vi "Init AI.vi"(8 "error in (no error)":errorcluster, 10 "ADC #":T1=-1, 11 "Session in":refnum<class "Session.lvclass">) -> (0 "error out":errorcluster, 3 "Session out":refnum<class "Session.lvclass">)   [LabVIEW 2024, in "CTI.lvlib" / "Session.lvclass"]
uses:
  Session.lvclass
  ADC Number.ctl
  DeviceComms/DeviceComms.lvclass
  CTI.lvlib
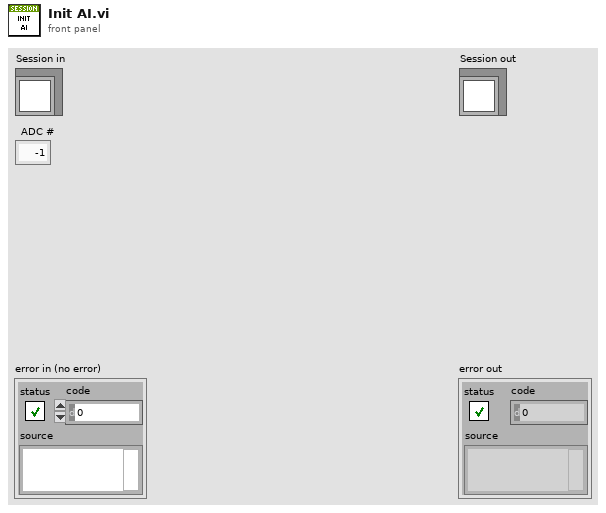
[diagram p1: front panel]
types:
  T1 = typedef "CTI.lvlib/ADC Number.ctl" = i8
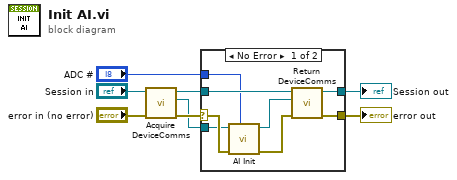
[diagram p0: block diagram]
diagram:
  n1 = call "Acquire DeviceComms.vi"("error in (no error)"="error in (no error)", "Session in"="Session in") -> ("error out"=w8:errorcluster, "DeviceComms"=w2:refnum<class "DeviceComms.lvclass">, "Session out"=w4:refnum<class "Session.lvclass">)  [unwired: 7 in]
  n2 = case shown="No Error" w8 {
    selector: w8 -> [w16 w18]
    tunnel: [w15 w18] -> w5
    tunnel: w4 -> [w14 w17]
    tunnel: [w13 w17] -> w3
    tunnel: w2 -> [w12 _]
    tunnel: "ADC #" -> [w11 _]
    frame No Error {
      n3 = call-dynamic "AI Init.vi"("ADC #"=w11, "error in (no error)"=w16, "DeviceComms in"=w12) -> ("error out"=w9:errorcluster, "DeviceComms out"=w10:refnum<class "DeviceComms.lvclass">)  [unwired: 7 in]
      n4 = call "Return DeviceComms.vi"("error in (no error)"=w9, "DeviceComms"=w10, "Session in"=w14) -> ("error out"=w15:errorcluster, "Session out"=w13:refnum<class "Session.lvclass">)  [unwired: 7 in]
    }
    frame Error {
    }
  }
  "error out" <- w5
  "Session out" <- w3
